vi "Time step.vi"(0 "Time (s)":dbl, 5 "Microwave on":bool=TRUE, 7 "Internal parameters in":T4, 9 "Fit parameters":T1, 11 "Physical constants":T3, 12 "System parameters":T2) -> (4 "Internal parameters out":T4, 15 "Fit parameters out":T1={"A"=0.572086, "S"=0.0835606, "M1"=140.286, "M2"=140.486})   [LabVIEW 2019]
uses:
  Internal Parameters.ctl
  Physical Constants.ctl
  System parameters.ctl
  Fit Parameters.ctl
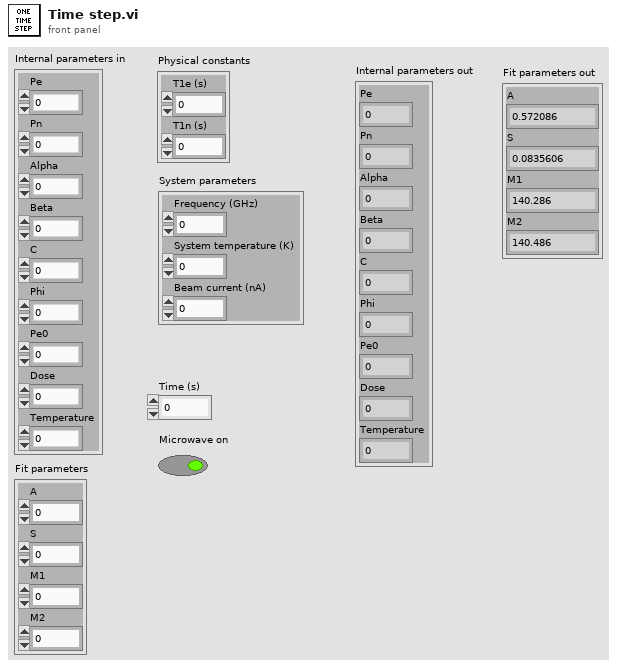
[diagram p1: front panel]
types:
  T1 = typedef "Fit Parameters.ctl" = cluster{"A":dbl, "S":dbl, "M1":dbl, "M2":dbl}
  T2 = typedef "System parameters.ctl" = cluster{"Frequency (GHz)":dbl, "System temperature (K)":dbl, "Beam current (nA)":dbl}
  T3 = typedef "Physical Constants.ctl" = cluster{"T1e (s)":dbl, "T1n (s)":dbl}
  T4 = typedef "Internal Parameters.ctl" = cluster{"Pe":dbl, "Pn":dbl, "Alpha":dbl, "Beta":dbl, "C":dbl, "Phi":dbl, "Pe0":dbl, "Dose":dbl, "Temperature":dbl}
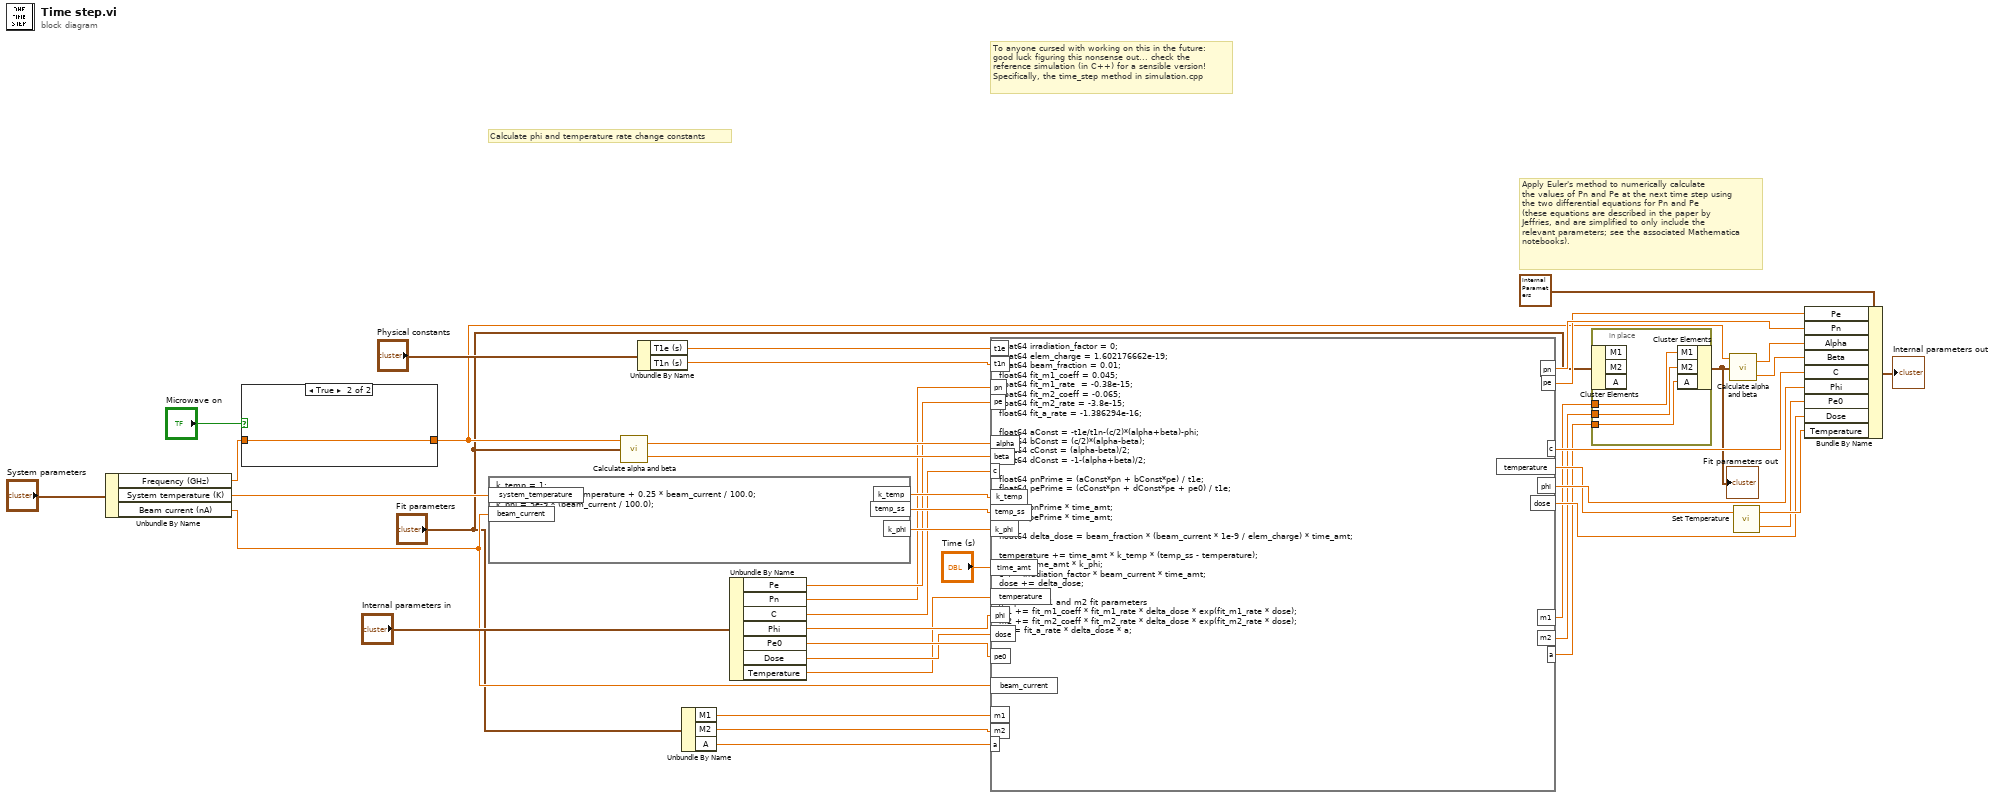
[diagram p0: block diagram]
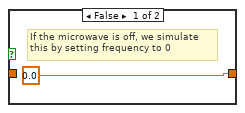
[diagram p2: hidden frame]
diagram:
  # "To anyone cursed with working on this in the future:\ngood luck figuring this nonsense out... check the\nreference simulation (in C++) for a sensible version!\nSpecifically, the time_step method in simulation.cpp"
  # "Apply Euler's method to numerically calculate\nthe values of Pn and Pe at the next time step using\nthe two differential equations for Pn and Pe\n(these equations are described in the paper by\nJeffries, and are simplified to only include the\nrelevant parameters; see the associated Mathematica\nnotebooks)."
  # "Calculate phi and temperature rate change constants"
  n1 = Unbundle By Name("System parameters") -> ("Frequency (GHz)"=w11:dbl, "System temperature (K)"=w34:dbl, "Beam current (nA)"=w24:dbl)
  n2 = case shown="True" "Microwave on" {
    tunnel: w11 -> [_ w45]
    tunnel: [0.0 ("Frequency") w45] -> w10
    frame False {
      # "If the microwave is off, we simulate\nthis by setting frequency to 0"
    }
    frame True {
    }
  }
  n3 = formula code="k_temp = 1;\ntemp_ss = system_temperature + 0.25 * beam_current / 100.0;\nk_phi = 5e-9 * (beam_current / 100.0);"("system_temperature"=w34, "beam_current"=w24) -> ("k_temp"=w43:dbl, "temp_ss"=w42:dbl, "k_phi"=w41:dbl)
  n4 = call "Calculate alpha and beta.vi"("Fit parameters"="Fit parameters", "Frequency (GHz)"=w10) -> ("Beta"=w39:dbl, "Alpha"=w40:dbl)  [unwired: 1 in]
  n5 = Unbundle By Name("Physical constants") -> ("T1e (s)"=w33:dbl, "T1n (s)"=w32:dbl)
  n6 = Unbundle By Name("Fit parameters") -> ("M1"=w8:dbl, "M2"=w7:dbl, "A"=w2:dbl)
  n7 = Unbundle By Name("Internal parameters in") -> ("Pe"=w31:dbl, "Pn"=w30:dbl, "C"=w29:dbl, "Phi"=w26:dbl, "Pe0"=w28:dbl, "Dose"=w27:dbl, "Temperature"=w25:dbl)
  n8 = formula code="float64 irradiation_factor = 0;\nfloat64 elem_charge = 1.602176662e-19;\nfloat64 beam_fraction = 0.01;\nfloat64 fit_m1_coeff = 0.045;\nfloat64 fit_m1_rate  = -0.38e-15;\nfloat64 fit_m2_coeff = -0.065;\nfloat64 fit_m2_rate = -3.8e-15;\nfloat64 fit_a_rate = -1.386294e-16;\n\nfloat64 aConst = -t1e/t1n-(c/2)*(alpha+beta)-phi;\nfloat64 bConst = (c/2)*(alpha-beta);\nfloat64 cConst = (alpha-beta)/2;\nfloat64 dConst = -1-(alpha+beta)/2;\n\nfloat64 pnPrime = (aConst*pn + bConst*pe) / t1e;\nfloat64 pePrime = (cConst*pn + dConst*pe + pe0) / t1e;\n\npn += pnPrime * time_amt;\npe += pePrime * time_amt;\n\nfloat64 delta_dose = beam_fraction * (beam_current * 1e-9 / elem_charge) * time_amt;\n\ntemperature += time_amt * k_temp * (temp_ss - temperature);\nphi += time_amt * k_phi;\nc += irradiation_factor * beam_current * time_amt;\ndose += delta_dose;\n\n// Update m1 and m2 fit parameters\nm1 += fit_m1_coeff * fit_m1_rate * delta_dose * exp(fit_m1_rate * dose);\nm2 += fit_m2_coeff * fit_m2_rate * delta_dose * exp(fit_m2_rate * dose);\na += fit_a_rate * delta_dose * a;"("pn"=w30, "pe"=w31, "t1e"=w33, "alpha"=w40, "beta"=w39, "c"=w29, "t1n"=w32, "k_temp"=w43, "temp_ss"=w42, "k_phi"=w41, "temperature"=w25, "time_amt"="Time (s)", "phi"=w26, "dose"=w27, "pe0"=w28, "beam_current"=w24, "m1"=w8, "m2"=w7, "a"=w2) -> ("pn"=w14:dbl, "pe"=w13:dbl, "temperature"=w9:dbl, "phi"=w18:dbl, "dose"=w20:dbl, "c"=w17:dbl, "m1"=w5:dbl, "m2"=w4:dbl, "a"=w1:dbl)
  n9 = in-place {
    in-place-border: w5 -> [w48]
    in-place-border: w4 -> [w47]
    in-place-border: w1 -> [w46]
    n10 = in-place-cluster #1("Fit parameters") -> ()  [unwired: 3 out]
    n11 = in-place-cluster #1("M1"=w48, "M2"=w47, "A"=w46) -> (w3:T1)
  }
  "Fit parameters out" <- w3
  n12 = call "Calculate alpha and beta.vi"("Fit parameters"=w3, "Frequency (GHz)"=w10) -> ("Beta"=w15:dbl, "Alpha"=w16:dbl)  [unwired: 1 in]
  n13 = call "Set Temperature.vi"("Temperature in"=w9) -> ("Pe0 out"=w19:dbl, "Temperature out"=w21:dbl)  [unwired: 1 in]
  n14 = Bundle By Name(cluster=T4 {"Pe"=0.0, "Pn"=0.0, "Alpha"=0.0, "Beta"=0.0, "C"=0.0, "Phi"=0.0, "Pe0"=0.0, "Dose"=0.0, "Temperature"=0.0} ("Simulation parameters out"), "Pe"=w13, "Pn"=w14, "Alpha"=w16, "Beta"=w15, "C"=w17, "Phi"=w18, "Pe0"=w19, "Dose"=w20, "Temperature"=w21) -> (→"Internal parameters out":T4)
